vi "Cut_Zero_Rows(Displacements)-1.vi"(1 "# Cols":i32, 2 "# Rows":i32, 3 "Array IN":dbl[][](array[numeric])) -> (0 "Array OUT":dbl[][](array[numeric]))   [LabVIEW 2013]
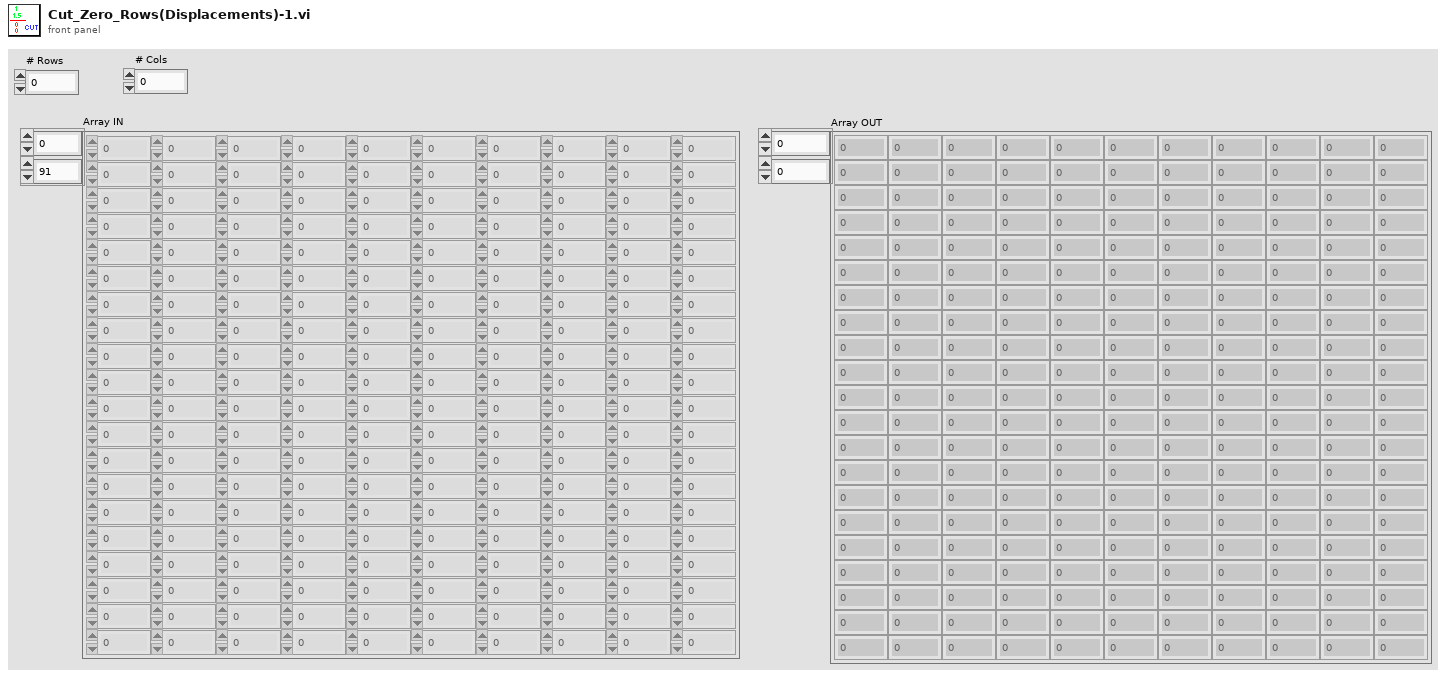
[diagram p1: front panel]
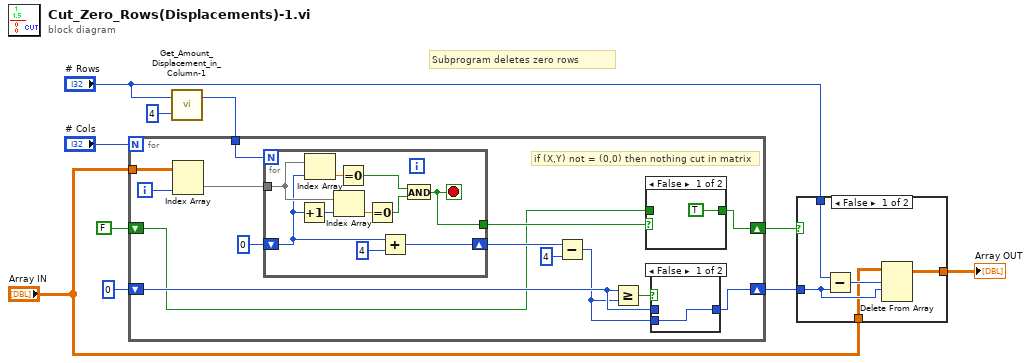
[diagram p0: block diagram]
diagram:
  # "Subprogram deletes zero rows"
  n1 = call "Get_Amount_Displacement_in_Column-1.vi"("multiplier"=4 ("y"), "# Rows"="# Rows") -> ("Displ amount"=w1:i32)  [unwired: 1 out]
  n2 = for {
    N: "# Cols" -> [_]
    tunnel: "Array IN" -> [w24]
    shift-right: [w12] -> w9
    shift-left: 0 -> [w19]
    shift-right: [w13] -> w4
    shift-left: FALSE -> [w14]
    tunnel: w1 -> [w11]
    i -> [w23]
    # "if (X,Y) not = (0,0) then nothing cut in matrix"
    n3 = Index Array(array=w24, index (col)=w23) -> (element=w22:dbl[])  [unwired: 1 in]
    n4 = for {
      N: w11 -> [_]
      tunnel: w22 -> [w34]
      shift-right: [w36] -> w18
      shift-left: 0 -> [w30]
      tunnel: [w29] -> w15
      stop <- w29 stop-if-true
      n5 = Increment(x=w30) -> (x+1=w35:i32)
      n6 = Index Array(array=w34, index=w30) -> (element=w38:dbl)
      n7 = Index Array(array=w34, index=w35) -> (element=w33:dbl)
      n8 = Equal To 0?(x=w38) -> (x = 0?=w32:bool)
      n9 = Equal To 0?(x=w33) -> (x = 0?=w31:bool)
      n10 = Add(x=w30, y=4) -> (x+y=w36:i32)
      n11 = And(x=w32, y=w31) -> (x .and. y?=w29:bool)
    }
    n12 = Subtract(x=w18, y=4) -> (x-y=w16:i32)
    n13 = Greater Or Equal?(x=w19, y=w16) -> (x >= y?=w20:bool)
    n14 = case shown="False" w15 {
      tunnel: w14 -> [_ w26]
      tunnel: [TRUE w26] -> w13
      frame False {
      }
      frame True {
      }
    }
    n15 = case shown="False" w20 {
      tunnel: w19 -> [_ w28]
      tunnel: [w27 w28] -> w12
      tunnel: w16 -> [w27 _]
      frame False {
      }
      frame True {
      }
    }
  }
  n16 = case shown="False" w4 {
    tunnel: w9 -> [w42 _]
    tunnel: [w41 w44] -> w8
    tunnel: "# Rows" -> [w40 _]
    tunnel: "Array IN" -> [w39 w44]
    frame False {
      n17 = Subtract(x=w40, y=w42) -> (x-y=w43:i32)
      n18 = Delete From Array(array=w39, length=w43, index (row)=w42) -> (array with subset deleted=w41:dbl[][])  [unwired: 1 in, 1 out]
    }
    frame True {
    }
  }
  "Array OUT" <- w8
